vi "Serialize.vi"(8 "error in (no error)":errorcluster, 11 "FrontPanelConverter in":refnum<class "FrontPanelConverter.lvclass">) -> (0 "error out":errorcluster, 2 "JSON":string, 3 "FrontPanelConverter out":refnum<class "FrontPanelConverter.lvclass">)   [LabVIEW 2017, in "FrontPanelConverter.lvclass"]
uses:
  FrontPanelConverter.lvclass
  <vilib>/Utility/miscctls.llb/LVRectTypeDef.ctl
  GObjectTypes.ctl
  JSONConstants.vi
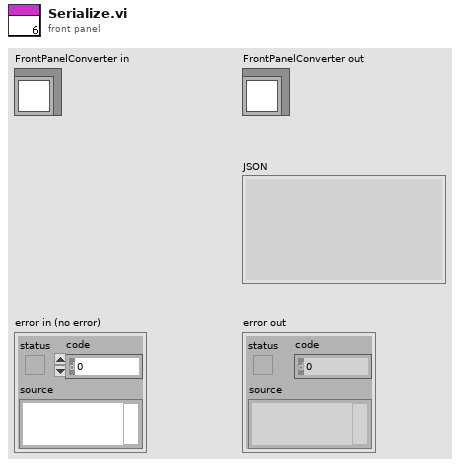
[diagram p1: front panel]
types:
  T1 = typedef "GObjectTypes.ctl" = enum16{"Diagram", "Panel"}
  T2 = typedef "LVRectTypeDef.ctl" = cluster{"Left":i16, "Top":i16, "Right":i16, "Bottom":i16}
  T3 = typedef "imagedata.ctl" = cluster{"image type":i32, "image depth":i32, "image":u8[], "mask":u8[], "colors":u32[], "Rectangle":cluster{"left":i16, "top":i16, "right":i16, "bottom":i16}}
  T4 = cluster{"left":i16, "top":i16, "right":i16, "bottom":i16}
  T5 = typedef "LVBoundsTypeDef.ctl" = cluster{"Width":u32, "Height":u32}
  T6 = typedef "LVPositionTypeDef.ctl" = cluster{"Left":i32, "Top":i32}
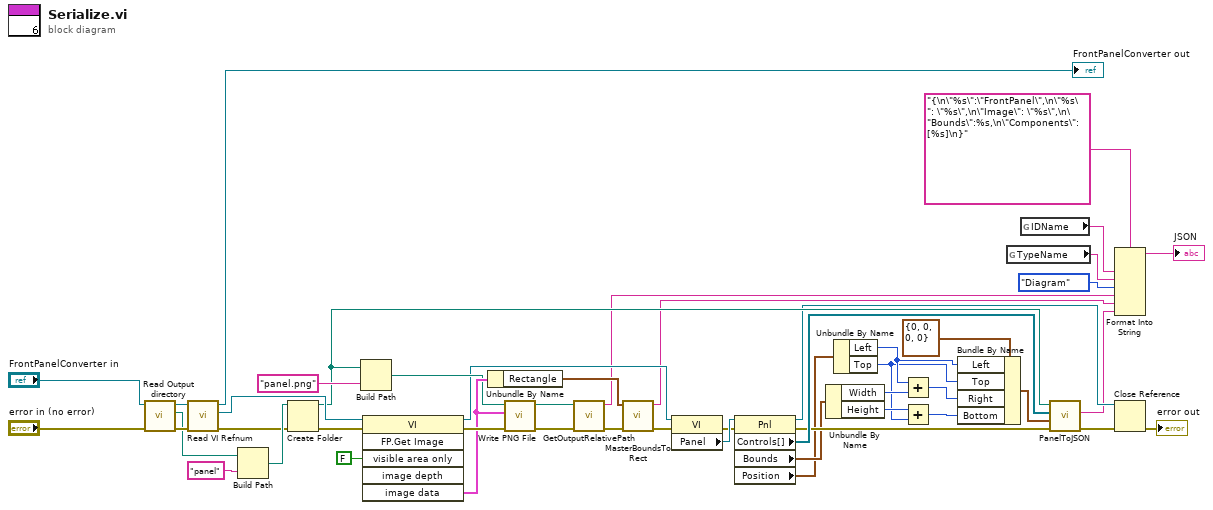
[diagram p0: block diagram]
diagram:
  n1 = call-dynamic "Read Output directory.vi"("error in (no error)"="error in (no error)", "GObjectConverterBase in"="FrontPanelConverter in") -> ("error out"=w30:errorcluster, "Output directory"=w20:path, "GObjectConverterBase out"=w46:refnum<class "FrontPanelConverter.lvclass">)  [unwired: 7 in]
  n2 = call-dynamic "Read VI Refnum.vi"("error in (no error)"=w30, "VIObjectConverter in"=w46) -> ("error out"=w19:errorcluster, "VI Refnum"=w18:refnum<vi>, "VIObjectConverter out"=→"FrontPanelConverter out":refnum<class "FrontPanelConverter.lvclass">)  [unwired: 7 in]
  n3 = Build Path(base path=w20, name or relative path="panel" ("string")) -> (appended path=w23:path)
  n4 = Create Folder(path (use dialog)=w23, error in=w19) -> (created path=w17:path, error out=w28:errorcluster)  [unwired: 1 in, 1 out]
  n5 = Build Path(base path=w17, name or relative path="panel.png" ("string")) -> (appended path=w21:path)
  n6 = invoke class="VI" method="FP.Get Image"(reference=w18, error in=w28, "visible area only"=FALSE ("Visible Area Only")) -> (reference out=w15:refnum<vi>, error out=w27:errorcluster, "image data"=w25:T3)  [unwired: 3 in, 3 out]
  n7 = Unbundle By Name(w25) -> ("Rectangle"=w16:T4)
  n8 = call <vilib>:"Write PNG File.vi"("error in (no error)"=w27, "image data"=w25, "path to PNG file"=w21) -> ("error out"=w10:errorcluster, "path"=w11:path)  [unwired: 7 in]
  n9 = call "GetOutputRelativePath.vi"("error in (no error)"=w10, "Path"=w11) -> ("error out"=w9:errorcluster, "Output relative path"=w4:string)  [unwired: 8 in]
  n10 = call "MasterBoundsToRect.vi"("error in"=w9, "Owner Bounds"=w16) -> ("error out"=w43:errorcluster, "JSON"=w3:string)  [unwired: 8 in]
  n11 = property class="VI"(reference=w15, error in=w43) -> (error out=w42:errorcluster, "Panel"=w45:refnum<vi>)  [unwired: 1 out]
  n12 = property class="Pnl"(reference=w45, error in=w42) -> (reference out=w14:refnum<vi>, error out=w41:errorcluster, "Controls[]"=w44:refnum<vi>[], "Bounds"=w40:T5, "Position"=w39:T6)
  n13 = Unbundle By Name(w40) -> ("Width"=w35:u32, "Height"=w33:u32)
  n14 = Unbundle By Name(w39) -> ("Left"=w36:i32, "Top"=w32:i32)
  n15 = Add(x=w36, y=w35) -> (x+y=w34:u32)
  n16 = Add(x=w33, y=w32) -> (x+y=w31:u32)
  n17 = Bundle By Name(cluster=T2 {"Left"=0, "Top"=0, "Right"=0, "Bottom"=0} ("Owner Bounds"), "Left"=w36, "Top"=w32, "Right"=w34, "Bottom"=w31) -> (w37:T2)
  n18 = global read "JSONConstants.vi" "TypeName"() -> (w6:string)
  n19 = global read "JSONConstants.vi" "IDName"() -> (w8:string)
  n20 = call "PanelToJSON.vi"("error in (no error)"=w41, "Owner Bounds"=w37, "Controls[]"=w44, "Folder Path"=w17) -> ("error out"=w12:errorcluster, "spreadsheet string"=w2:string)  [unwired: 6 in]
  n21 = Format Into String(format string="{\n\"%s\":\"FrontPanel\",\n\"%s\": \"%s\",\n\"Image\": \"%s\",\n\"Bounds\":%s,\n\"Components\": [%s]\n}", w8, w6, GObjectTypes."Diagram" ("GObject Types"), w4, w3, w2) -> (resulting string=→"JSON":string)  [unwired: 2 in, 1 out]
  n22 = Close Reference(reference=w14, error in (no error)=w12) -> (error out=→"error out":errorcluster)
